vi "initialise task.vi"(8 "error in (no error)":errorcluster, 11 "ImagingModeSPIM in":refnum<class "ImagingModeSPIM.lvclass">) -> (0 "error out":errorcluster, 3 "ImagingModeSPIM out":refnum<class "ImagingModeSPIM.lvclass">)   [LabVIEW 2012, in "ImagingModeSPIM.lvclass"]
uses:
  ImagingModeSPIM.lvclass
  ImagingModeSPIM.lvclass/ImagingModeSPIM.ctl
  <vilib>/DAQmx/create/channels.llb/DAQmx Create Channel (AO-Voltage-Basic).vi
  <vilib>/DAQmx/write.llb/DAQmx Write (Analog DBL 1Chan 1Samp).vi
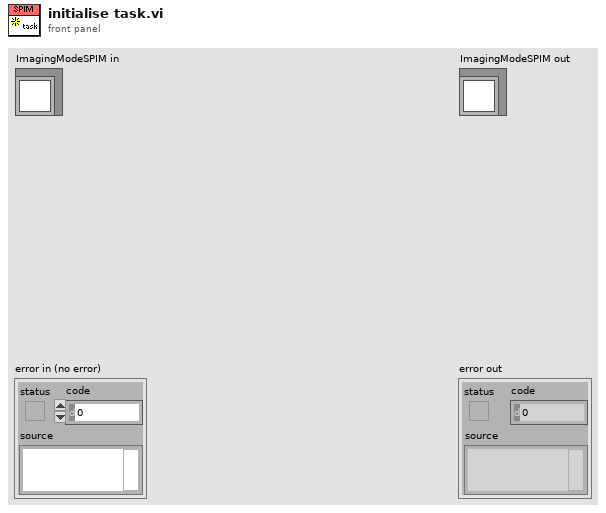
[diagram p1: front panel]
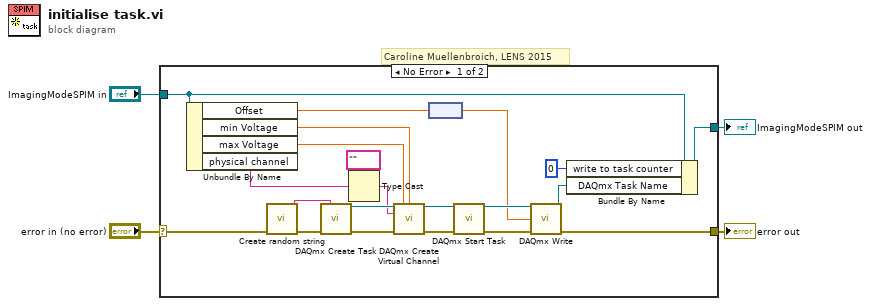
[diagram p0: block diagram]
diagram:
  # "Caroline Muellenbroich, LENS 2015"
  n1 = case shown="No Error" "error in (no error)" {
    selector: "error in (no error)" -> [w7 w27]
    tunnel: [w14 w27] -> w3
    tunnel: [w24 w26] -> w1
    tunnel: "ImagingModeSPIM in" -> [w25 w26]
    frame No Error {
      n2 = Unbundle By Name(w25) -> ("Offset"=w13:dbl[unit], "min Voltage"=w22:dbl, "max Voltage"=w23:dbl, "physical channel"=w21:string)
      n3 = call "Create random string.vi"("error in"=w7) -> ("error out"=w6:errorcluster, "string"=w5:string)  [unwired: 9 in]
      n4 = call <vilib>:"DAQmx Create Task.vi"("new task name"=w5, "error in"=w6) -> ("task out"=w10:refnum<k21>, "error out"=w11:errorcluster)  [unwired: 12 in]
      n5 = Type Cast(type=tag "" ("physical channels"), x=w21) -> (*(type *) &x=w8:tag)
      n6 = call-poly <vilib>:"DAQmx Create Virtual Channel.vi"("task in"=w10, "maximum value"=w23, "minimum value"=w22, "physical channels"=w8, "error in"=w11) -> ("task out"=w18:refnum<k21>, "error out"=w20:errorcluster)  [unwired: 9 in]
      n7 = node(w13) -> (w12:dbl)
      n8 = call <vilib>:"DAQmx Start Task.vi"("task/channels in"=w18, "error in"=w20) -> ("task out"=w15:refnum<k21>, "error out"=w16:errorcluster)  [unwired: 12 in]
      n9 = call-poly <vilib>:"DAQmx Write.vi"("task/channels in"=w15, "data"=w12, "error in"=w16) -> ("task out"=w17:refnum<k21>, "error out"=w14:errorcluster)  [unwired: 10 in, 1 out]
      n10 = Bundle By Name(cluster=w25, "write to task counter"=0 ("runtime cluster.Task cluster.write to task counter"), "DAQmx Task Name"=w17) -> (w24:refnum<class "ImagingModeSPIM.lvclass">)
    }
    frame Error {
    }
  }
  "error out" <- w3
  "ImagingModeSPIM out" <- w1
